vi "Measurement Parser old.vi"(8 "error in (no error)":errorcluster, 9 "Generic Card in":refnum<class "Generic Card.lvclass">, 10 "Data Array":dbl[](array[numeric]), 11 "Tektronix PA1000 in":refnum<class "Tektronix PA1000.lvclass">) -> (3 "Tektronix PA1000 out":refnum<class "Tektronix PA1000.lvclass">)   [LabVIEW 2014]
uses:
  Tektronix PA1000.lvclass
  Generic Instrument/Generic Card/Generic Card.lvclass
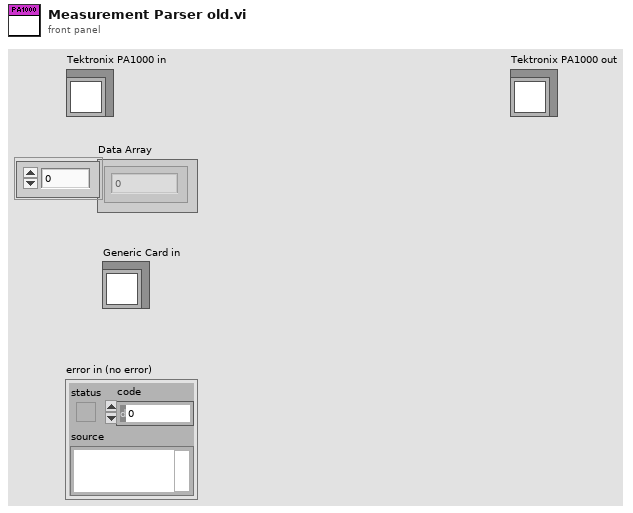
[diagram p1: front panel]
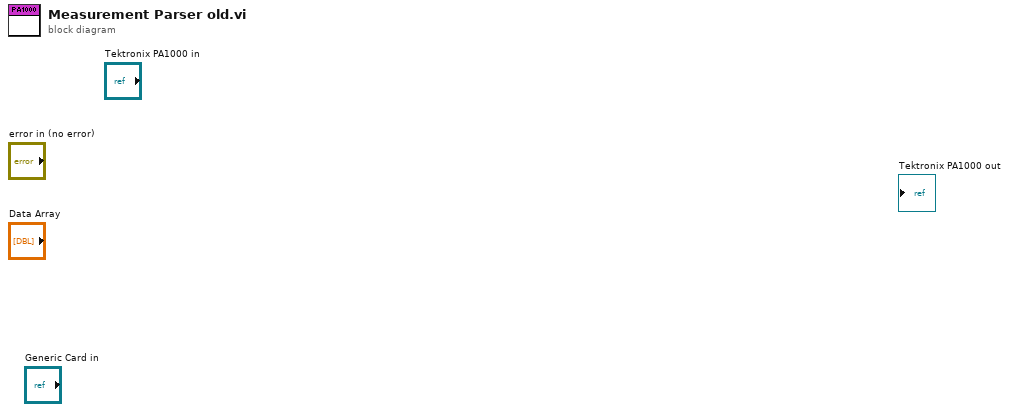
[diagram p0: block diagram]
diagram:
